vi "Projecte 2.0.vi"() -> ()   [LabVIEW 2014]
uses:
  <vilib>/Instr/_visa.llb/VISA Find Search Mode.ctl
  <vilib>/Utility/file.llb/Write To Spreadsheet File (I64).vi
panel:
  out "XY Graph":cluster{i32[], i32[]}(graph)
  out "lectura":i32[](array[numeric])=[49, 49, 49, 49, 49, 49, 49, 49, 49, 49, 49, 49, 49, 49, 49, 49, 49, 48, 48, 49, 49, 49, 49, 49, 49, 48, 49, 49, 48, 49, 49, 49, 49, 49, 49, 49, 48, 49, 49, 48, 48, 48, 48, 49, 49, 48, 49, 49, 49, 48, 49, 49, 49, 49, 48, 49, 48, 49, 49, 49, 48, 48, 49, 49, 48, 48, 48, 48, 48, 48, 48, 49, 49, 49, 49, 48, 49, 49, 49, 49, 49, 49, 49, 49, 48, 49, 49, 49, 49, 49, 48, 48, 48, 48, 48, 49, 49, 49, 49, 49, 49, 49, 49, 48, 49, 49, 48, 49, 49, 48, 49, 49, 48, 49, 49, 48, 48, 48, 49, 48, 49, 49, 49, 49, 48, 48, 49, 48, 48, 49, 49, 48, 49, 49, 49, 49, 48, 49, 49, 49, 48, 49, 48, 48, 48, 48, 48, 49, 49, 49, 48, 48, 48, 49, 49, 49, 48, 48, 49, 48, 48, 49, 49, 49, 48, 49, 48, 48, 48, 48, 49, 48, 49, 49, 48, 49, 49, 49, 49, 48, 48, 48, 49, 48, 49, 49, 49, 48, 49, 48, 182, 194, 203, 203, 202, 202, 203, 203, 203, 203, 203, 203, 203, 203, 203, 204, 204, 204, 203, 203, 204, 204, 204, 204, 204, 204, 204, 204, 204, 204, 204, 204, 204, 204, 205, 204, 204, 205, 204, 204, 204, 205, 205, 205, 205, 205, 205, 205, 204, 205, 205, 205, 204, 206, 205, 205, 205, 205, 205, 205, 205, 206, 206, 206, 205, 205, 206, 206, 206, 205, 206, 206, 206, 207, 206, 205, 206, 206, 206, 206, 206, 206, 206, 206, 206, 206, 206, 206, 206, 206, 206, 207, 206, 207, 207, 207, 207, 207, 206, 207, 207, 207, 206, 206, 206, 207, 206, 206, 207, 207, 207, 207, 207, 207, 207, 206, 207, 208, 207, 207, 208, 207, 207, 207, 207, 207, 207, 207, 207, 207, 207, 207, 207, 207, 207, 207, 207, 207, 207, 207, 207, 207, 207, 207, 207, 207, 208, 207, 207, 207, 208, 207, 207, 207, 207, 207, 208, 207, 207, 207, 208, 207, 208, 208, 207, 207, 207, 208, 207, 207, 207, 207, 208, 207, 207, 208, 208, 208, 208, 208, 208, 208, 208, 208, 208, 208, 208, 208, 207, 208, 208, 208, 207, 208, 208, 208, 208, 208, 208, 208, 208, 208, 209, 207, 208, 207, 207, 208, 208, 207, 207, 208, 207, 208, 207, 208, 208, 208, 208, 208, 208, 208, 208, 208, 208, 208, 208, 208, 208, 208, 208, 208, 208, 208, 208, 208, 207, 208, 208, 208, 208, 208, 208, 208, 208, 208, 209, 208, 208, 208, 209, 209, 208, 208, 208, 207, 208, 208, 208, 208, 208, 208, 208, 208, 208, 208, 208, 208, 209, 208, 208, 208, 208, 208, 208, 208, 208, 208, 208, 208, 208, 209, 208, 208, 208, 208, 208, 208, 208, 208, 209, 208, 208, 208, 208, 208, 208, 208, 208, 208, 208, 209, 208, 208, 208, 208, 208, 209, 208, 208, 209, 208, 209, 208, 208, 208, 208, 209, 208, 208, 208, 208, 209, 208, 208, 208, 208, 208, 208, 209, 209, 208, 208, 208, 209, 208, 208, 208, 208, 208, 208, 209, 208, 208, 208, 208, 209, 208, 208, 208, 208, 208, 209, 208, 208, 208, 208, 208, 208, 208, 208, 208, 208, 208, 209, 208, 209, 208, 208, 208, 209, 208, 208, 208, 208, 208, 209, 209, 208, 208, 209, 208, 209, 208, 208, 208, 209, 208, 209, 209, 209, 208, 209, 208, 209, 208, 208, 209, 208, 209, 209, 209, 209, 209, 209, 183, 69, 56, 54, 54, 54, 54, 54, 54, 54, 53, 53, 53, 54, 53, 54, 53, 53, 54, 53, 53, 53, 53, 53, 53, 53, 53, 52, 53, 53, 52, 53, 53, 53, 53, 52, 52, 53, 52, 52, 52, 52, 53, 52, 52, 52, 51, 53, 52, 52, 52, 52, 52, 52, 52, 51, 51, 51, 52, 51, 51, 51, 52, 51, 52, 51, 51, 51, 51, 51, 51, 51, 51, 51, 51, 50, 51, 51, 51, 51, 51, 51, 51, 50, 50, 50, 50, 51, 50, 50, 50, 50, 51, 49, 50, 50, 51, 50, 50, 50, 50, 51, 50, 50, 50, 50, 50, 50, 50, 49, 50, 50, 50, 50, 50, 50, 50, 50, 49, 50, 50, 50, 50, 50, 50, 50, 50, 50, 49, 50, 50, 50, 49, 50, 49, 49, 50, 50, 49, 50, 49, 49, 49, 50, 49, 50, 50, 49, 49, 49, 50, 49, 49, 49, 50, 49, 49, 49, 49, 49, 50, 49, 49, 49, 49, 49, 49, 49, 49, 50, 49, 49, 49, 49, 49, 49, 49, 49, 49, 49, 50, 49, 49, 49, 49, 49, 49, 49, 49, 49, 48, 49, 49, 49, 48, 49, 49, 49, 49, 49, 49, 49, 49, 49, 49, 49, 49, 49, 48, 49, 49, 48, 49, 48, 49, 49, 50, 48, 49, 49, 49, 49, 49, 49, 49, 49, 48, 49, 48, 49, 48, 49, 49, 48, 49, 49, 49, 49, 48, 49, 50, 49, 48, 49, 49, 49, 48, 49, 49, 49, 49, 48, 49, 49, 49, 48, 48, 48, 48, 48, 48, 49, 49, 48, 49, 49, 48, 49, 49, 48, 49, 49, 49, 49, 49, 49, 49, 49, 48, 48, 48, 48, 48, 49, 48, 48, 49, 49, 49, 49, 49, 48, 48, 48, 49, 49, 49, 48, 49, 49, 48, 49, 49, 49, 49, 49, 48, 48, 48, 48, 48, 48, 48, 48, 48, 48, 48, 49, 48, 49, 48, 48, 48, 48, 48, 49, 49, 49, 49, 48, 49, 49, 49, 48, 49, 49, 49, 49, 48, 48, 48, 48, 48, 48, 49, 48, 49, 48, 48, 49, 48, 48, 48, 49, 49, 49, 48, 48, 48, 48, 48, 48, 49, 49, 48, 49, 48, 49, 49, 48, 49, 49, 48, 49, 48, 48, 49, 49, 48, 48, 49, 49, 49, 48, 48, 48, 48, 49, 49, 49, 48, 48, 48, 49, 48, 48, 48, 48, 49, 48, 48, 48, 49, 49, 48, 48, 174, 190, 203, 203, 202, 202, 202, 203, 203, 203, 203, 203, 203, 203, 203, 203, 203, 203, 204, 203, 204, 203, 203, 203, 203, 204, 204, 204, 204, 204, 204, 204, 204, 203, 204, 204, 204, 205, 205, 205, 205, 204, 205, 204, 205, 204, 205, 205, 205, 205, 205, 205, 205, 205, 205, 205, 205, 205, 205, 205, 206, 205, 206, 206, 206, 206, 205, 206, 206, 205, 205, 206, 205, 206, 206, 206, 206, 206, 206, 206, 206, 206, 206, 206, 206, 206, 207, 206, 207, 206, 206, 207, 206, 207, 206, 207, 207, 206, 206, 207, 207, 207, 207, 206, 207, 206, 206, 206, 207, 207, 207, 207, 207, 206, 207, 206, 207, 207, 207, 207, 207, 207, 206, 207, 207, 207, 207, 207, 207, 207, 207, 207, 207, 207, 207, 207, 207, 208, 207, 207, 207, 207, 208, 208, 207, 207, 207, 207, 207, 207, 207, 207, 207, 207, 207, 207, 207, 207, 207, 207, 207, 208, 208, 207, 207, 207, 207, 207, 208, 208, 207, 207, 207, 207, 207, 208, 207, 207, 207, 208, 208, 208, 208, 207, 208, 208, 207, 208, 208, 208, 208, 208, 208, 208, 208, 208, 208, 207, 207, 208, 208, 208, 208, 208, 207, 208, 207, 208, 207, 208, 207, 208, 208, 209, 208, 208, 208, 208, 208, 208, 207, 208, 208, 208, 208, 208, 208, 208, 208, 208, 208, 208, 208, 208, 208, 208, 208, 208, 208, 208, 208, 208, 208, 208, 208, 208, 208, 208, 208, 208, 208, 208, 208, 209, 208, 208, 208, 208, 208, 208, 208, 208, 208, 208, 208, 208, 208, 208, 208, 208, 208, 208, 207, 208, 208, 208, 208, 208, 208, 208, 208, 209, 208, 208, 208, 208, 209, 208, 208, 208, 208, 208, 209, 208, 209, 208, 208, 209, 208, 208, 209, 209, 208, 209, 208, 208, 208, 208, 208, 208, 209, 208, 209, 208, 208, 208, 208, 209, 209, 208, 208, 208, 208, 208, 208, 208, 208, 209, 209, 208, 208, 208, 208, 208, 208, 208, 208, 209, 208, 208, 209, 208, 208, 209, 208, 208, 208, 208, 208, 208, 208, 208, 208, 208, 208, 209, 209, 208, 208, 208, 208, 208, 208, 209, 208, 208, 208, 208, 208, 208, 209, 209, 209, 209, 208, 209, 208, 209, 209, 209, 208, 209, 209, 209, 208, 208, 208, 208, 208, 208, 208, 208, 208, 208, 208, 208, 208, 209, 208, 208, 208, 208, 208, 208, 208, 208, 99, 56, 54, 54, 54, 54, 54, 54, 54, 54, 54, 53, 54, 53, 54, 54, 53, 53, 53, 54, 54, 53, 53, 53, 53, 53, 53, 52, 52, 52, 52, 53, 52, 53, 53, 52, 53, 52, 53, 52, 52, 52, 52, 52, 52, 51, 52, 52, 52, 52, 51, 51, 51, 51, 51, 52, 51, 51, 51, 51, 52, 51, 51, 51, 52, 51, 51, 51, 51, 51, 51, 51, 51, 51, 50, 51, 51, 51, 51, 51, 51, 51, 51, 51, 51, 51, 51, 51, 51, 51, 50, 51, 50, 50, 50, 50, 50, 51, 50, 50, 50, 50, 50, 50, 50, 50, 49, 50, 50, 50, 50, 50, 50, 50, 51, 50, 50, 50, 50, 49, 50, 49, 50, 50, 50, 50, 50, 50, 49, 50, 49, 50, 50, 50, 50, 50, 50, 50, 50, 50, 49, 49, 49, 50, 49, 49, 49, 49, 50, 50, 50, 50, 49, 49, 49, 49, 49, 49, 49, 49, 49, 50, 49, 49, 49, 49, 50, 49, 49, 49, 49, 49, 49, 49, 49, 49, 49, 49, 49, 49, 49, 49, 49, 50, 49, 49, 49, 49, 49, 49, 50, 49, 49, 49, 49, 49, 50, 49, 49, 49, 49, 49, 48, 49, 49, 48, 49, 49, 49, 49, 49, 50, 49, 49, 49, 49, 49, 49, 49, 49, 49, 49, 49, 48, 48, 49, 49, 49, 49, 49, 49, 49, 49, 49, 49, 50, 49, 49, 49, 49, 49, 49, 49, 49, 49, 48, 49, 48, 49, 49, 49, 48, 49, 48, 48, 49, 49, 49, 48, 49, 49, 49, 49, 49, 48, 49, 49, 48, 48, 49, 49, 49, 49, 48, 48, 48, 48, 48, 48, 49, 49, 48, 49, 49, 48, 49, 49, 49, 49, 48, 49, 49, 49, 49, 48, 49, 48, 48, 49, 48, 48, 48, 48, 49, 49, 48, 49, 48, 48, 48, 48, 48, 48, 48, 49, 49, 49, 49, 48, 48, 49, 49, 48, 49, 48, 48, 48, 48, 48, 49, 49, 48, 48, 49, 49, 49, 48, 49, 48, 48, 49, 48, 49, 49, 49, 48, 49, 48, 49, 48, 48, 48, 48, 49, 48, 48, 48, 49, 48, 48, 48, 49, 48, 49, 48, 48, 49, 48, 49, 49, 49, 48, 48, 48, 48, 48, 48, 49, 48, 48, 49, 49, 49, 48, 49, 48, 48, 49, 48, 48, 49, 48, 49, 48, 48, 49, 49, 48, 49, 48, 48, 48, 49, 48, 49, 71, 182, 202, 202, 202, 203, 202, 202, 203, 203, 203, 203, 204, 203, 203, 203, 203, 203, 204, 203, 204, 204, 203, 203, 203, 204, 204, 204, 204, 205, 204, 204, 204, 204, 204, 204, 204, 204, 204, 205, 205, 205, 205, 204, 205, 205, 205, 205, 205, 205, 205, 204, 205, 205, 205, 205, 205, 205, 205, 205, 205, 205, 206, 205, 206, 205, 205, 206, 206, 206, 206, 206, 206, 206, 206, 206, 206, 206, 206, 206, 206, 206, 206, 206, 206, 206, 206, 206, 207, 207, 207, 206, 206, 206, 205, 207, 207, 206, 206, 206, 207, 207, 206, 206, 206, 206, 207, 206, 207, 206, 207, 207, 207, 207, 207, 207, 207, 207, 207, 207, 207, 207, 207, 207, 207, 207, 207, 207, 207, 207, 207, 207, 208, 207, 207, 207, 207, 207, 207, 207, 207, 207, 207, 208, 207, 207, 207, 207, 207, 207, 207, 208, 207, 207, 207, 207, 208, 207, 207, 207, 208, 207, 207, 207, 207, 207, 207, 207, 207, 208, 208, 207, 208, 207, 208, 207, 208, 207, 208, 207, 207, 208, 208, 208, 208, 207, 208, 208]
  in  "access (0:read/write)":enum16{"read/write", "read-only", "write-only"}(ring)=enum."write-only"
  in  "operation (0:open)":T1(ring)=enum."replace or create"
  in  "file path (use dialog)":path=path "E:/prova.txt"
  in  "nuum del aparell":i32
  out "llista d 'aparells":string[](array[string])=["GPIB0::7::INSTR"]
  in  "Search Mode":T2 items=["Canonical Names Only"=0, "Aliases Only"=2, "Include Matching Aliases"=3, "Include All Aliases"=4]
  in  "expression (\"?*\")":string="GPIB?*INSTR"
  out "Instrument":string="HEWLETT-PACKARD,54603B,0,1.2\n"
  out "error out":errorcluster
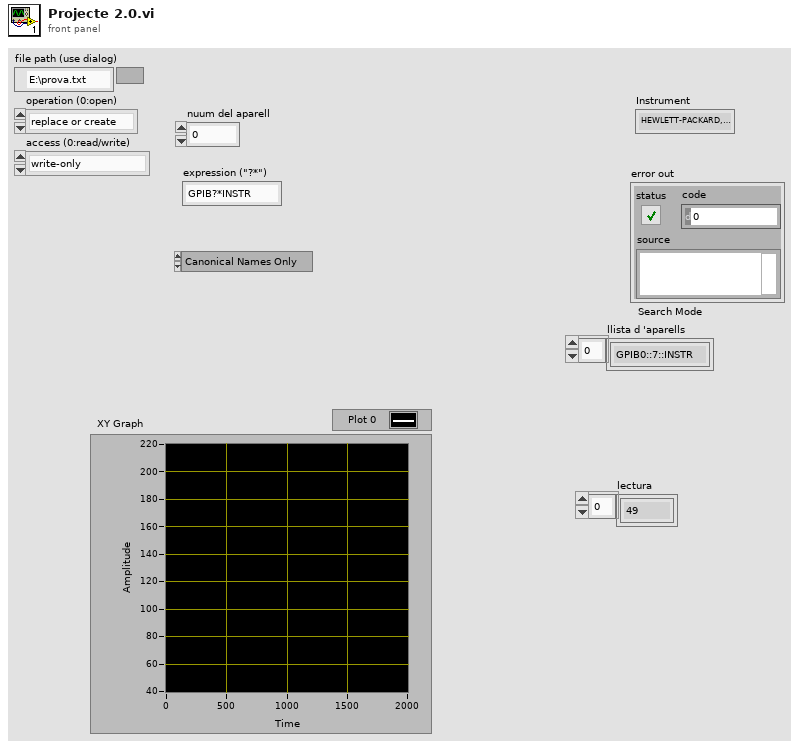
[diagram p1: front panel]
types:
  T1 = enum16{"open", "replace", "create", "open or create", "replace or create", "replace or create with confirmation"}
  T2 = typedef "VISA Find Search Mode.ctl" = u32
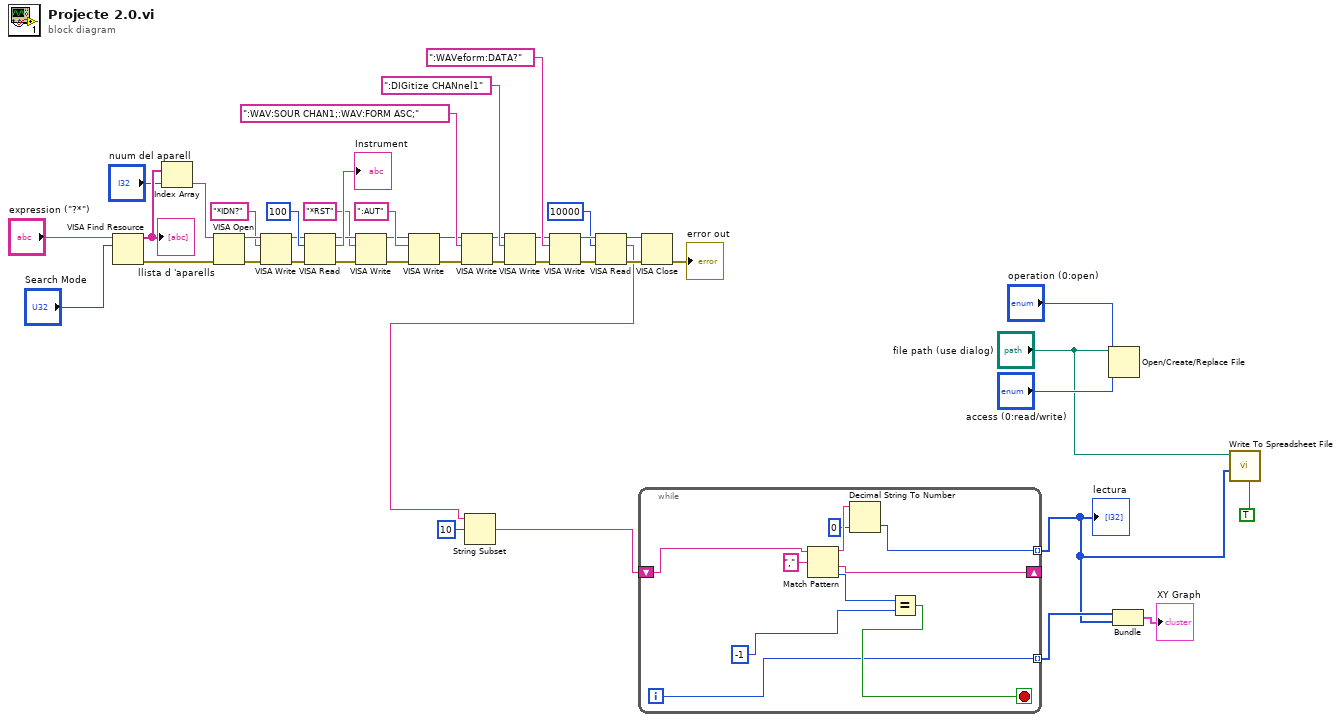
[diagram p0: block diagram]
diagram:
  n1 = VISA Find Resource(10:"Search Mode", 11:"expression (\"?*\")") -> (0:w37:errorcluster, 3:w34:string[])  [unwired: 1 in, 1 out]
  "llista d 'aparells" <- w34
  n2 = Index Array(array=w34, index="nuum del aparell") -> (element=w32:string)
  n3 = VISA Open(error in (no error)=w37, VISA resource name=w32) -> (VISA resource name=w44:refnum<visa-resource-name>, error out=w43:errorcluster)  [unwired: 3 in]
  n4 = VISA Write(VISA resource name=w44, write buffer="*IDN?", error in (no error)=w43) -> (VISA resource name out=w31:refnum<visa-resource-name>, error out=w42:errorcluster)  [unwired: 1 out]
  n5 = VISA Read(VISA resource name=w31, byte count=u32 100, error in (no error)=w42) -> (VISA resource name out=w30:refnum<visa-resource-name>, read buffer=→"Instrument":string, error out=w29:errorcluster)  [unwired: 1 out]
  n6 = VISA Write(VISA resource name=w30, write buffer="*RST", error in (no error)=w29) -> (VISA resource name out=w19:refnum<visa-resource-name>, error out=w18:errorcluster)  [unwired: 1 out]
  n7 = VISA Write(VISA resource name=w19, write buffer=":AUT", error in (no error)=w18) -> (VISA resource name out=w17:refnum<visa-resource-name>, error out=w16:errorcluster)  [unwired: 1 out]
  n8 = VISA Write(VISA resource name=w17, write buffer=":WAV:SOUR CHAN1;:WAV:FORM ASC;", error in (no error)=w16) -> (VISA resource name out=w15:refnum<visa-resource-name>, error out=w14:errorcluster)  [unwired: 1 out]
  n9 = VISA Write(VISA resource name=w15, write buffer=":DIGitize CHANnel1", error in (no error)=w14) -> (VISA resource name out=w13:refnum<visa-resource-name>, error out=w12:errorcluster)  [unwired: 1 out]
  n10 = VISA Write(VISA resource name=w13, write buffer=":WAVeform:DATA?", error in (no error)=w12) -> (VISA resource name out=w26:refnum<visa-resource-name>, error out=w25:errorcluster)  [unwired: 1 out]
  n11 = VISA Read(VISA resource name=w26, byte count=u32 10000, error in (no error)=w25) -> (VISA resource name out=w20:refnum<visa-resource-name>, read buffer=w5:string, error out=w9:errorcluster)  [unwired: 1 out]
  n12 = String Subset(string=w5, offset (0)=10) -> (substring=w3:string)  [unwired: 1 in]
  n13 = while {
    shift-right: [w52] -> _
    shift-left: w3 -> [w53]
    tunnel: [w47] -> w6 mode=indexing
    tunnel: [w45] -> w8 mode=indexing
    i -> [w45]
    stop <- w49 stop-if-true
    n14 = Match Pattern(string=w53, regular expression=",") -> (before substring=w48:string, after substring=w52:string, offset past match=w51:i32)  [unwired: 1 in, 1 out]
    n15 = Decimal String To Number(string=w48, default (0L)=0 ("default (0 I32)")) -> (number=w47:i32)  [unwired: 1 in, 1 out]
    n16 = Equal?(x=w51, y=-1) -> (x = y?=w49:bool)
  }
  "lectura" <- w6
  n17 = VISA Close(VISA resource name=w20, error in (no error)=w9) -> (error out=→"error out":errorcluster)
  n18 = Open/Create/Replace File(file path (use dialog)="file path (use dialog)", operation (0:open)="operation (0:open)", access (0:read/write)="access (0:read/write)") -> ()  [unwired: 3 in, 3 out]
  n19 = Bundle(w8, w6) -> (→"XY Graph":cluster{i32[], i32[]})  [unwired: 1 in]
  n20 = call-poly <vilib>:"Write To Spreadsheet File.vi"("transpose? (no:F)"=TRUE, "1D data"=w6, "file path (dialog if empty)"="file path (use dialog)") -> ()  [unwired: 5 in, 1 out]
